vi "Test.vi"(11 "Command Line Arguments":string[](array[string])) -> (2 "test details":string, 3 "Exit Code":i32)   [LabVIEW 2017]
uses:
  <vilib>/addons/_JKI.lib/_jki_lib_vi_tester_junit_xml_results.llb/TextTestRunner.JUnitXML.lvclass
  C:/Program Files/National Instruments/LabVIEW 2017/vi.lib/addons/_JKI Toolkits/VI Tester/TextTestRunner.llb/TextTestRunner.lvclass
  <vilib>/addons/_JKI Toolkits/VI Tester/VI Tester API.llb/Run Tests (Path Array).vi
  <vilib>/addons/_JKI Toolkits/VI Tester/VI Tester API.llb/VI Tester API.lvlib
  C:/Program Files/National Instruments/LabVIEW 2017/vi.lib/addons/_JKI Toolkits/VI Tester/TestRunner.llb/TestRunner.lvclass
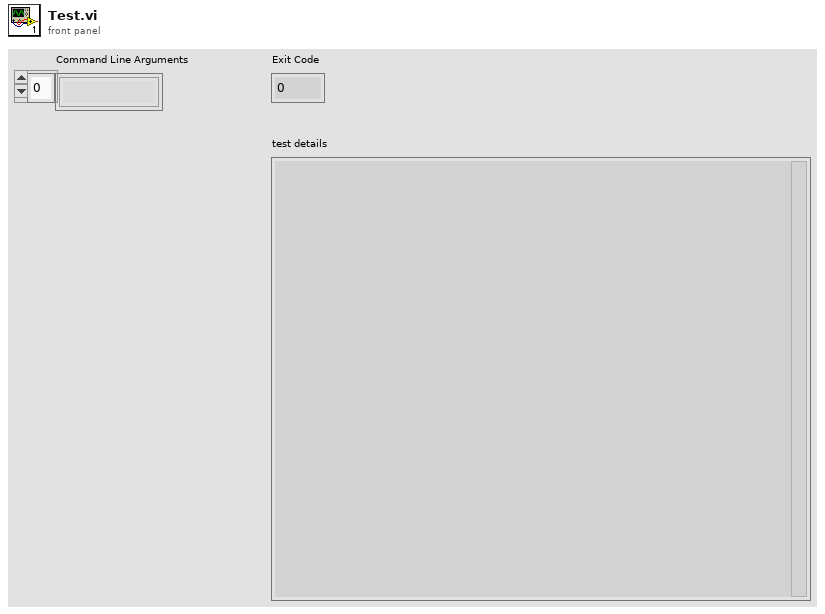
[diagram p1: front panel]
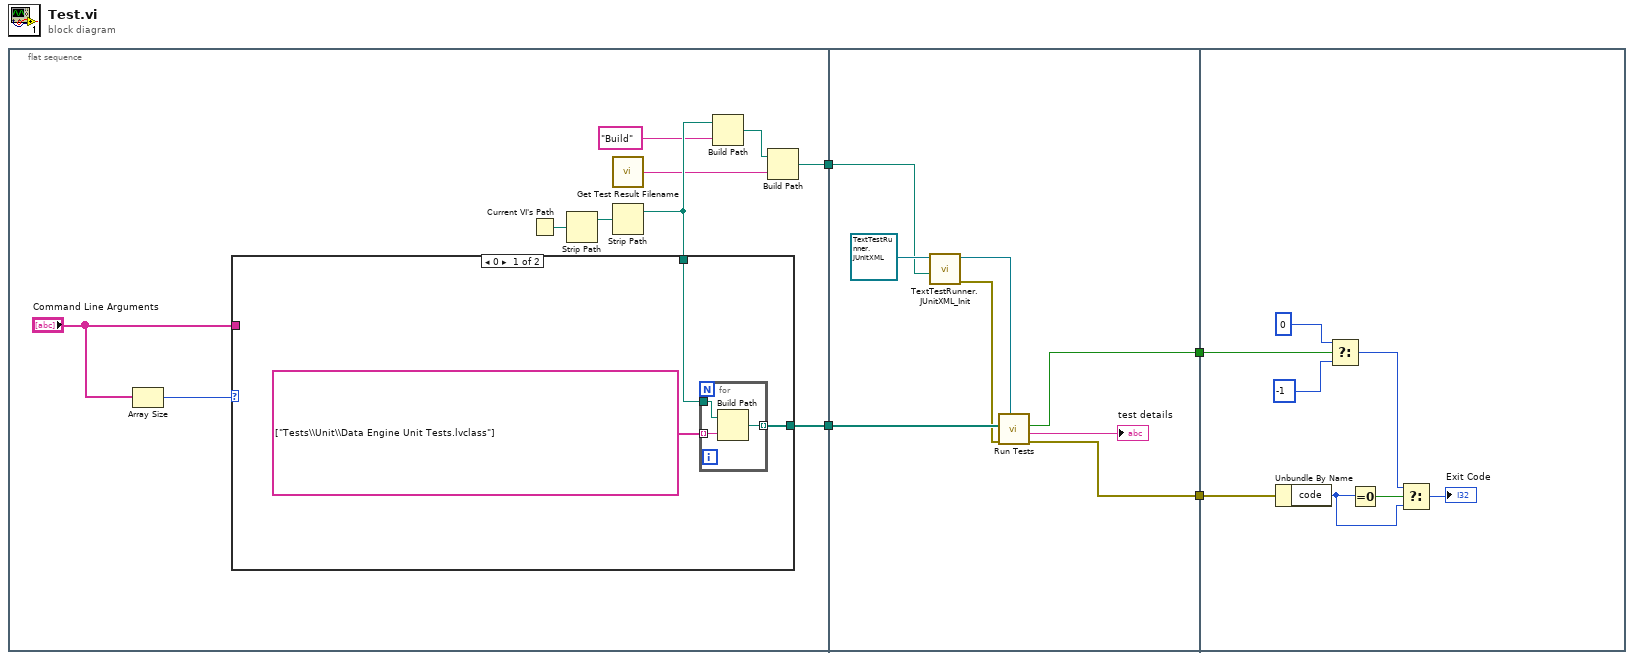
[diagram p0: block diagram]
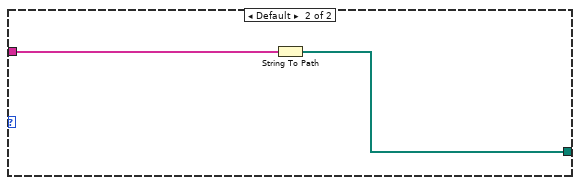
[diagram p2: hidden frame]
diagram:
  n1 = flat-sequence {
    tunnel: [w14] -> w4
    tunnel: [w5] -> w1
    tunnel: w4 -> [w29]
    tunnel: [w27] -> w3
    tunnel: [w28] -> w2
    tunnel: w1 -> [w24]
    tunnel: w3 -> [w35]
    tunnel: w2 -> [w38]
    frame #0 {
      n2 = Array Size(array="Command Line Arguments") -> (size(s)=w13:i32)
      n3 = Current VI's Path() -> (path=w11:path)
      n4 = Strip Path(path=w11) -> (stripped path=w10:path)  [unwired: 1 out]
      n5 = call "Get Test Result Filename.vi"() -> ("TestResult Filename out"=w7:string)
      n6 = Strip Path(path=w10) -> (stripped path=w9:path)  [unwired: 1 out]
      n7 = case shown="0" w13 {
        tunnel: [w16 w21] -> w14
        tunnel: "Command Line Arguments" -> [_ w22]
        tunnel: w9 -> [w15 _]
        frame 0 {
          n8 = for {
            tunnel: string[] ["Tests\\Unit\\Data Engine Unit Tests.lvclass"] -> [w20] mode=indexing
            tunnel: [w19] -> w16 mode=indexing
            tunnel: w15 -> [w18]
            n9 = Build Path(base path=w18, name or relative path=w20) -> (appended path=w19:path)
          }
        }
        frame Default {
          n10 = String To Path(string=w22) -> (path=w21:path[])
        }
      }
      n11 = Build Path(base path=w9, name or relative path="Build") -> (appended path=w8:path)
      n12 = Build Path(base path=w8, name or relative path=w7) -> (appended path=w5:path)
    }
    frame #1 {
      n13 = call <vilib>:"TextTestRunner.JUnitXML_Init.vi"("Report Path"=w24, "TextTestRunner in"=refnum<class "TextTestRunner.JUnitXML.lvclass"> refnum ("TextTestRunner.Ant.lvclass")) -> ("error out"=w23:errorcluster, "TextTestRunner out"=w25:refnum<class "TextTestRunner.JUnitXML.lvclass">)  [unwired: 8 in]
      n14 = call-poly <vilib>:"Run Tests.vi"("TextTestRunner in"=w25, "error in (no error)"=w23, "Test Paths"=w29) -> ("error out"=w27:errorcluster, "test details"=→"test details":string, "successful?"=w28:bool)  [unwired: 6 in]
    }
    frame #2 {
      n15 = Unbundle By Name(w35) -> ("code"=w32:i32)
      n16 = Select(t=0, s=w38, f=-1) -> (s? t:f=w33:i32)
      n17 = Equal To 0?(x=w32) -> (x = 0?=w34:bool)
      n18 = Select(t=w33, s=w34, f=w32) -> (s? t:f=→"Exit Code":i32)
    }
  }
